vi "CreatePrivateEvents.vi"(8 "error in (no error)":errorcluster, 11 "Instrument.Oxford1820":refnum<class "Instrument.Oxford1820.lvclass">) -> (0 "error out":errorcluster, 3 "Instrument.Oxford1820 out":refnum<class "Instrument.Oxford1820.lvclass">)   [LabVIEW 2019, in "Instrument.Oxford1820.lvclass"]
doc: "---------------------------------------------------------------\nJKI State Machine Objects™\nhttp://jki.net/state-machine-objects/\nCopyright (C) 2005-2015, JKI <info@jki.net>\nALL RIGHTS RESERVEDJKI State Machine Objects (SMO) 1.0.0.4\nJKI - JKI\nCopyright (c) 2015, JKI"
uses:
  Instrument.Oxford1820.lvclass
  Typedefs/PrivateEvents--Instrument.Oxford1820.SequenceSetMagnetField.ctl
  <userlib>/LevyLab/Instrument Framework/Instrument Types/Cryostat/Instrument.Cryostat.lvclass
  Typedefs/PrivateEvents--Instrument.Oxford1820.AbortSequence.ctl
  <userlib>/LevyLab/Instrument Framework/Instrument Types/Cryostat/Typedefs/Magnet Mode--Enum.ctl
  <userlib>/LevyLab/Instrument Framework/Instrument Types/Cryostat/Typedefs/Magnet Axis--Enum.ctl
  <userlib>/LevyLab/Instrument Framework/SMOs/RemoteControl/Typedefs/Message--Cluster.ctl
  <userlib>/LevyLab/Instrument Framework/SMOs/RemoteControl/RemoteControl.lvclass
  Typedefs/PrivateEvents--Instrument.Oxford1820.MessageToProcess.ctl
  Typedefs/PrivateEvents--Instrument.Oxford1820.setMagnetField.ctl
panel:
  # "For instructions on how to use the JKI State Machine Objects, examples and video tutorials, visit:\nhttp://jki.net/state-machine-objects/\n\nJKI State Machine Objects™\nhttp://jki.net/state-machine-objects/\nCopyright (C) 2005-2015, JKI <info@jki.net>\nALL RIGHTS RESERVED"
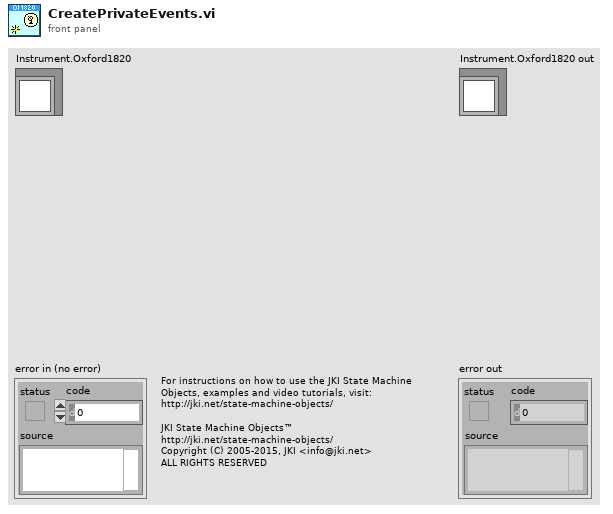
[diagram p1: front panel]
types:
  T1 = typedef "Instrument.Oxford1820.lvclass/PrivateEvents--Instrument.Oxford1820.MessageToProcess.ctl" = cluster{"Message":T2}
  T2 = typedef "RemoteControl.lvclass/Message--Cluster.ctl" = cluster{"Command":string, "Data":variant, "ID":string}
  T3 = typedef "Instrument.Oxford1820.lvclass/PrivateEvents--Instrument.Oxford1820.AbortSequence.ctl" = bool
  T4 = typedef "Instrument.Oxford1820.lvclass/PrivateEvents--Instrument.Oxford1820.SequenceSetMagnetField.ctl" = cluster{"setMagnetField":T5}
  T5 = typedef "Instrument.Oxford1820.lvclass/PrivateEvents--Instrument.Oxford1820.setMagnetField.ctl" = cluster{"field":dbl, "rate":dbl, "axis":T6, "mode":T7}
  T6 = typedef "Instrument.Cryostat.lvclass/Magnet Axis--Enum.ctl" = enum16{"Z", "X", "Y"}
  T7 = typedef "Instrument.Cryostat.lvclass/Magnet Mode--Enum.ctl" = enum16{"Persistent", "Driven"}
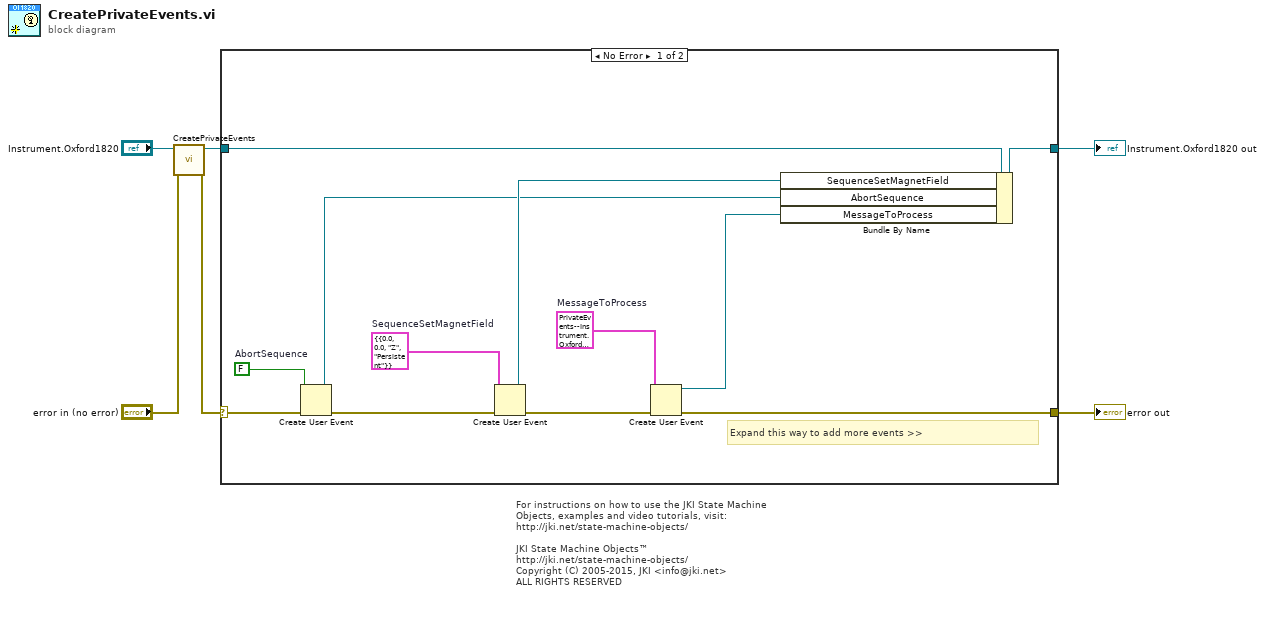
[diagram p0: block diagram]
diagram:
  # "For instructions on how to use the JKI State Machine Objects, examples and video tutorials, visit:\nhttp://jki.net/state-machine-objects/\n\nJKI State Machine Objects™\nhttp://jki.net/state-machine-objects/\nCopyright (C) 2005-2015, JKI <info@jki.net>\nALL RIGHTS RESERVED"
  n1 = call-parent "CreatePrivateEvents.vi"("error in (no error)"="error in (no error)", "Instrument"="Instrument.Oxford1820") -> ("error out"=w1:errorcluster, "Instrument out"=w3:refnum<class "Instrument.Oxford1820.lvclass">)  [unwired: 8 in]
  n2 = case shown="No Error" w1 {
    selector: w1 -> [w14 w20]
    tunnel: [w9 w20] -> w5
    tunnel: [w17 w19] -> w6
    tunnel: w3 -> [w18 w19]
    frame No Error {
      w8 = T1 {"Message"={"Command"="", "Data"=variant(string ""), "ID"=""}}  # MessageToProcess
      w12 = T3 FALSE  # AbortSequence
      w16 = T4 {"setMagnetField"={"field"=0.0, "rate"=0.0, "axis"=enum."Z", "mode"=enum."Persistent"}}  # SequenceSetMagnetField
      # "Expand this way to add more events >>"
      n3 = Create User Event(user event datatype=w12, error in=w14) -> (user event=w11:refnum<user-event>, error out=w13:errorcluster)
      n4 = Create User Event(user event datatype=w16, error in=w13) -> (user event=w15:refnum<user-event>, error out=w10:errorcluster)
      n5 = Create User Event(user event datatype=w8, error in=w10) -> (user event=w7:refnum<user-event>, error out=w9:errorcluster)
      n6 = Bundle By Name(cluster=w18, "SequenceSetMagnetField"=w15, "AbortSequence"=w11, "MessageToProcess"=w7) -> (w17:refnum<class "Instrument.Oxford1820.lvclass">)
    }
    frame Error {
    }
  }
  "error out" <- w5
  "Instrument.Oxford1820 out" <- w6
